vi "re_sig.confirm_lua.vi"(5 "LuaVIEW reference":T1) -> (15 "error out":errorcluster)   [LabVIEW 2012]
doc: "Sends a \"confirm\" signal to the specified task. Note that the purpose of waiting for a confirm signal is to give the operator a chance to review a task's error message. Programmatic confirmation, through calling this function, should therefore be done only as a last resort to force tasks that keep on hanging in error mode to terminate.\nParameters:\nstr:task_identifier\nResults:\nbool:signal_set"
uses:
  typedefs/t_LuaVIEW Reference.ctl
  typedefs/t_LuaVIEW Task List Methods.ctl
  subvis/private/LuaVIEW Push (boolean).vi
  subvis/private/LuaVIEW Pull (string).vi
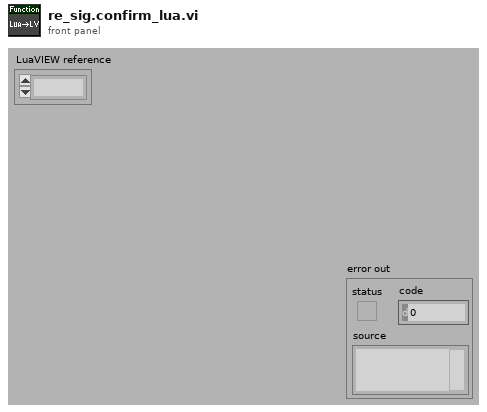
[diagram p1: front panel]
types:
  T1 = typedef "t_LuaVIEW Reference.ctl" = refnum<k1>
  T2 = typedef "t_LuaVIEW Task List Methods.ctl" = enum16{"clear list", "add", "test", "remove", "get ref", "get task info", "get list", "get script info", "ongoing?", "resume", "pause", "stop", "confirm", "message"}
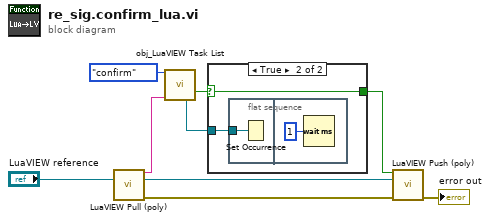
[diagram p0: block diagram]
diagram:
  n1 = call-poly "LuaVIEW Pull (poly).vi"("LuaVIEW reference in"="LuaVIEW reference") -> ("string"=w3:string, "LuaVIEW reference out"=w1:T1, "error out"=w2:errorcluster)  [unwired: 12 in]
  n2 = call "obj_LuaVIEW Task List.vi"("method"=t_LuaVIEW_Task_List_Methods."confirm", "task identifier"=w3) -> ("set/ongoing"=w8:bool, "wakeup occurrence"=w7:refnum<k4>)  [unwired: 8 in, 4 out]
  n3 = case shown="True" w8 {
    selector: w8 -> [w10 w12]
    tunnel: w7 -> [_ w11]
    tunnel: [w10 w12] -> w6
    frame False {
    }
    frame True {
      n4 = flat-sequence {
        tunnel: w11 -> [w13]
        frame #0 {
          n5 = Set Occurrence(w13) -> ()
        }
        frame #1 {
          n6 = Wait (ms)(milliseconds to wait=u32 1) -> ()  [unwired: 1 out]
        }
      }
    }
  }
  n7 = call-poly "LuaVIEW Push (poly).vi"("boolean"=w6, "LuaVIEW reference in"=w1, "error in (no error)"=w2) -> ("error out"=→"error out":errorcluster)  [unwired: 11 in, 1 out]
